vi "Z-Projection.vi"(8 "error in":errorcluster, 9 "[ROI vis]":T4 caption="[POI]" {"ROI number" min=1 format="ROI %.0f"}, 11 "Functional Imging UI Refs":T2) -> (0 "error out":errorcluster, 2 "GreenPOIMax":T1, 3 "RedPOIMax":T1)   [LabVIEW 2013]
uses:
  <vilib>/vision/Image Controls.llb/IMAQ Image.ctl
  Typedefs/ROI selector array-ROI vis.ctl
  xcontrol/Interface VIs/Interface typedefs/Interface-ROI selection cluster.ctl
  Typedefs/ROI ID Enum.ctl
  Typedefs/Functional Imging UI Refs.ctl
  xcontrol/XGrapher.xctl
  Typedefs/Groups array referecne.ctl
  Typedefs/ROI visibility mode.ctl
  Typedefs/Get-Set-Clear Control.ctl
  Typedefs/ROI parameters data type.ctl
  Global variables/gl_Functional Imaging-Global variables.vi
  <vilib>/vision/NI_Vision_Development_Module.lvlib
panel:
  out "Image 2":T1(plugin-control)
  out "Red norm max":i16
  out "Red max":i16
  out "Image":T1(plugin-control)
  out "Green norm max":i16
  in  "Normalise to approx.":i16=3000
  out "Green max":i16
  out "Multiple Z-planes added":bool
  # "[Groups] is a Typedef"
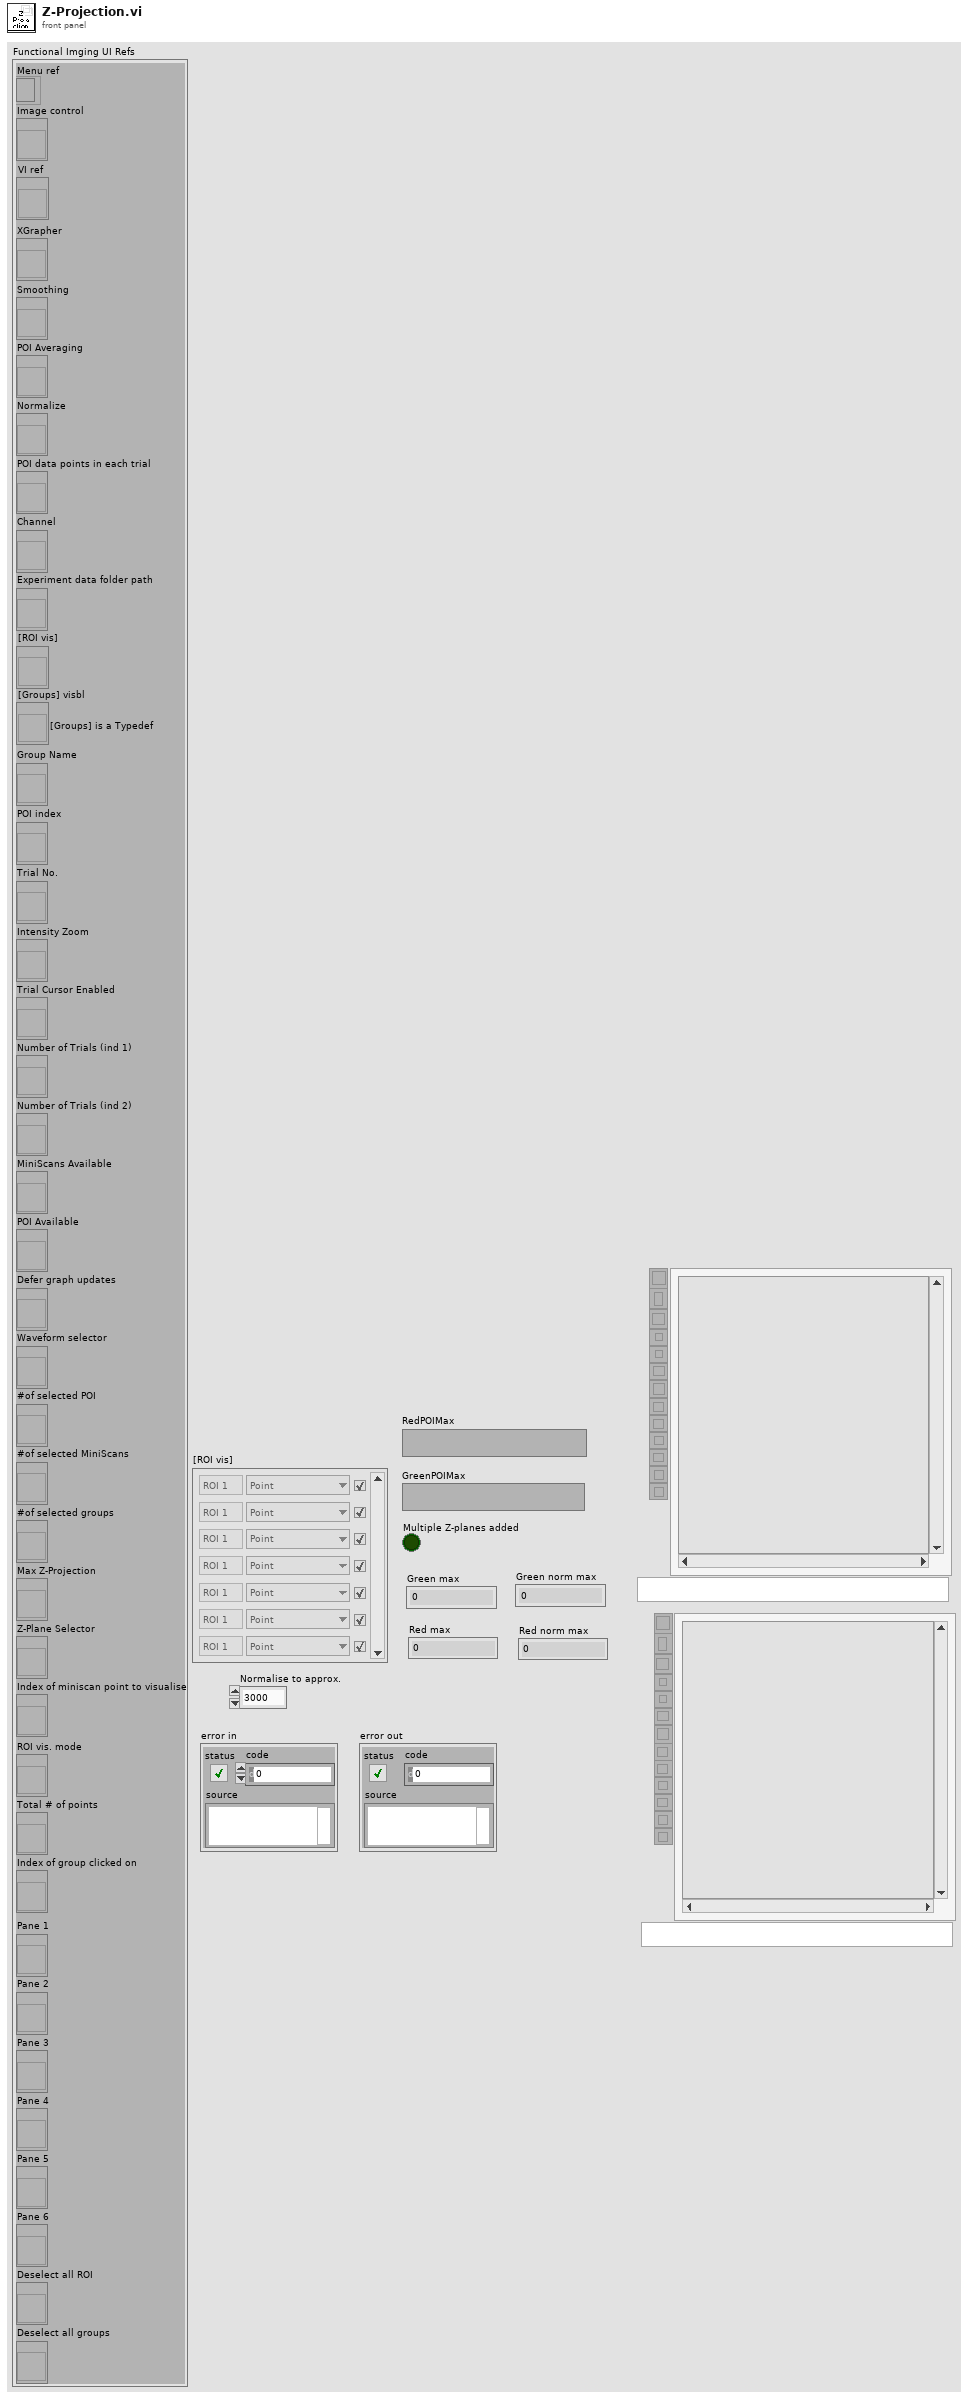
[diagram p1: front panel]
types:
  T1 = typedef "IMAQ Image.ctl" = refnum<image>
  T2 = typedef "Functional Imging UI Refs.ctl" = cluster{"Menu ref":refnum<k9>, "Image control":refnum<vi>, "VI ref":refnum<vi>, "XGrapher":refnum<vi>, "Smoothing":refnum<vi>, "POI Averaging":refnum<vi>, "Normalize":refnum<vi>, "POI data points in each trial":refnum<vi>, "Channel":refnum<vi>, "Experiment data folder path":refnum<vi>, "[ROI vis]":refnum<vi>, "[Groups] visbl":T3, "Group Name":refnum<vi>, "POI index":refnum<vi>, "Trial No.":refnum<vi>, "Intensity Zoom":refnum<vi>, "Trial Cursor Enabled":refnum<vi>, "Number of Trials (ind 1)":refnum<vi>, "Number of Trials (ind 2)":refnum<vi>, "MiniScans Available":refnum<vi>, "POI Available":refnum<vi>, "Defer graph updates":refnum<vi>, "Waveform selector":refnum<vi>, "#of selected POI":refnum<vi>, "#of selected MiniScans":refnum<vi>, "#of selected groups":refnum<vi>, "Max Z-Projection":refnum<vi>, "Z-Plane Selector":refnum<vi>, "Index of miniscan point to visualise":refnum<vi>, "ROI vis. mode":refnum<vi>, "Total # of points":refnum<vi>, "Index of group clicked on":refnum<vi>, "Pane 1":refnum<vi>, "Pane 2":refnum<vi>, "Pane 3":refnum<vi>, "Pane 4":refnum<vi>, "Pane 5":refnum<vi>, "Pane 6":refnum<vi>, "Deselect all ROI":refnum<vi>, "Deselect all groups":refnum<vi>}
  T3 = typedef "Groups array referecne.ctl" = refnum<vi>
  T4 = typedef "ROI selector array-ROI vis.ctl" = T5[]
  T5 = typedef "Interface-ROI selection cluster.ctl" = cluster{"ROI number":i32, "ROI ID":T6, "Visibility":bool}
  T6 = typedef "ROI ID Enum.ctl" = enum16{"Point", "MiniScan", "Comp. MiniScan", "Rectangle", "Comp. volume", "Arb. plane point"}
  T7 = typedef "Get-Set-Clear Control.ctl" = enum16{"Get", "Set", "Clear"}
  T8 = typedef "ROI parameters data type.ctl" = cluster{"ROI index":dbl, "ROI ID":dbl, "ROI Time (ns)":dbl, "Pixels in ROI":dbl, "X start":dbl, "Y start":dbl, "Z start":dbl, "X stop":dbl, "Y stop":dbl, "Z stop":dbl, "Angle (deg)":dbl, "Composite ID":dbl, "Number of lines":dbl, "Frame Size":dbl, "Zoom":dbl, "Laser Power (%)":dbl, "ROI group ID":dbl}
  T9 = enum32{"Average", "Min", "Max", "Clear  if < ", "Clear  if < or =", "Clear  if =", "Clear  if > or =", "Clear  if >"}
  T10 = typedef "Image Type" = u32
  T11 = typedef "Functional Parameters Cluster.ctl" = cluster{"ROI data":dbl[][], "ROI format version":i32, "Norm ROI data":dbl[][], "Norm. ROI format version":i32, "Z norm":dbl[], "Z norm format version":i32}
  T12 = typedef "Fixed strings.ctl" = cluster{"ROI file name":string, "Normalised ROI file name":string, "Zplane Pockels values file name":string, "Functional data folder name":string, "Experiment Header file name":string, "Z-stack images folder name":string, "Groups setup rel. path":string, "Groups text file rel. path":string, "TDMS files folder name (F.img)":string, "TDMS files folder name (V.acq)":string, "TDMS files folder name (Pl.acq)":string, "Cycle rel times sequence file":string, "Dynamically called VIs folder name":string, "Time Series folder base name":string}
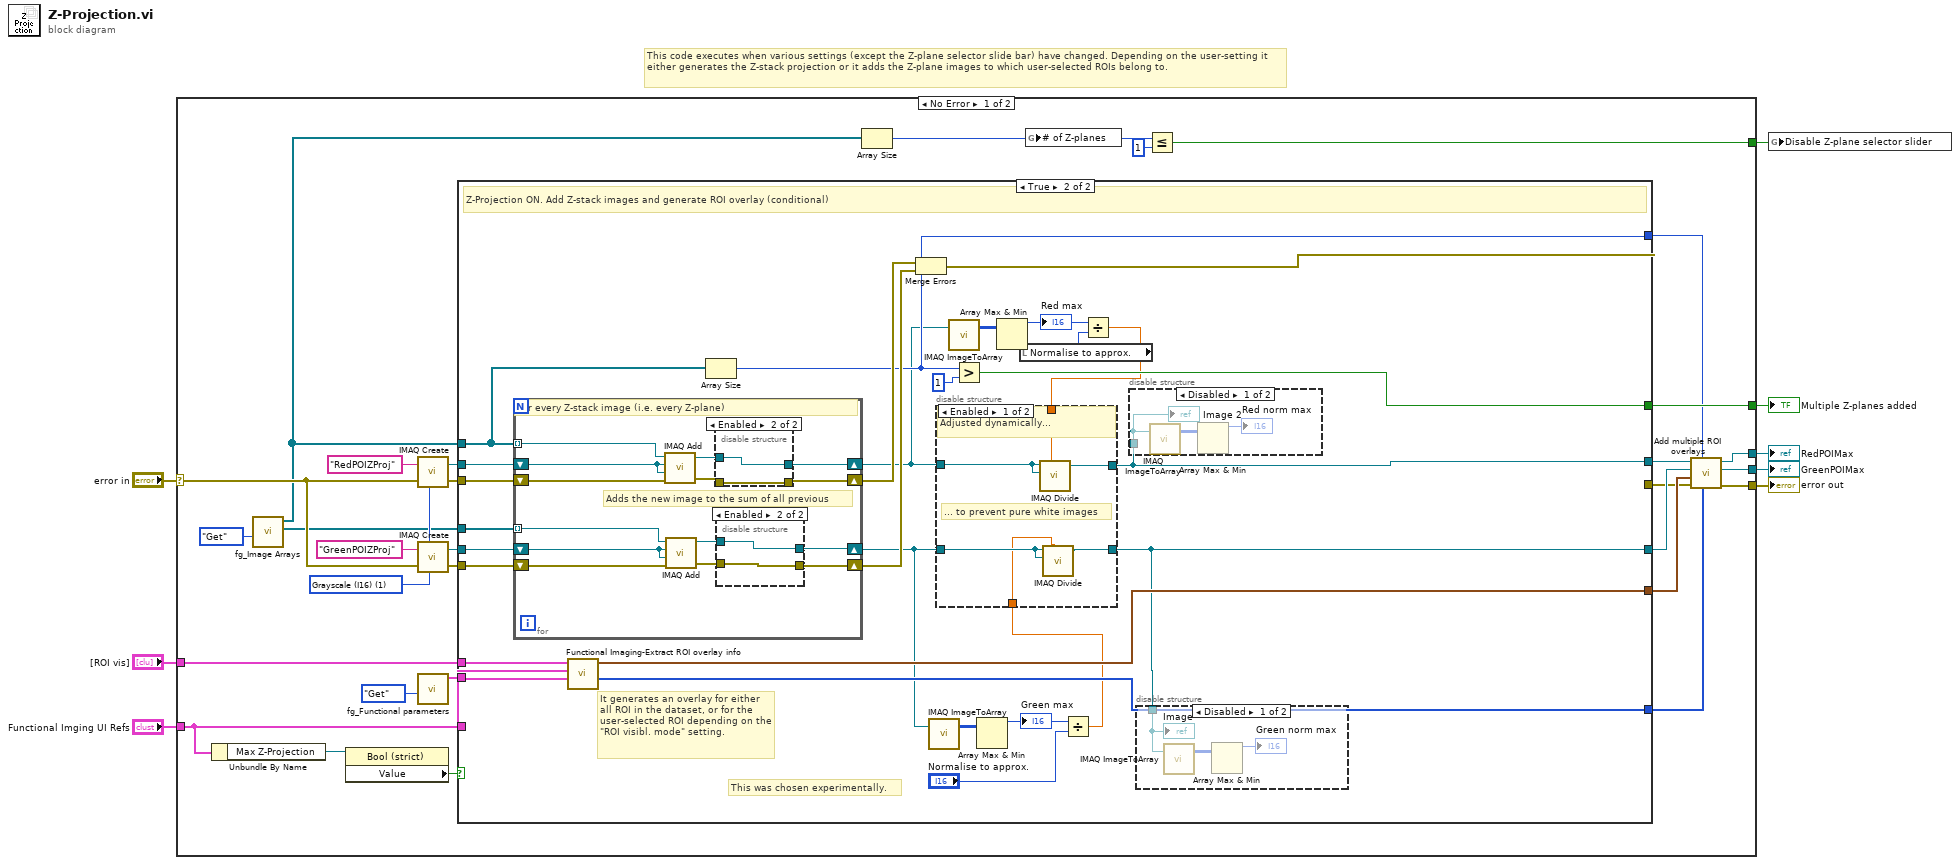
[diagram p0: block diagram]
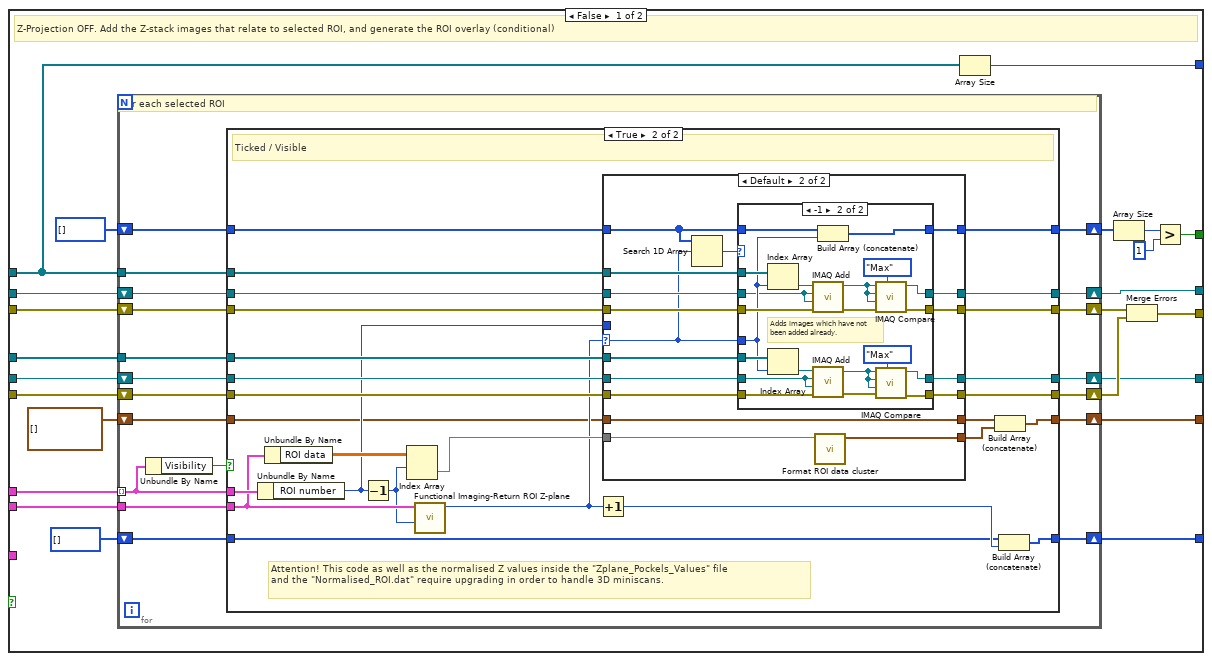
[diagram p2: hidden frame]
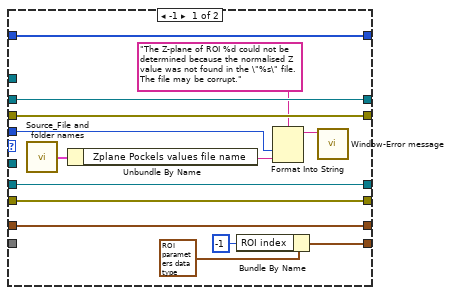
[diagram p4: hidden frame]
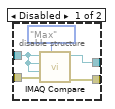
[diagram p9: hidden frame]
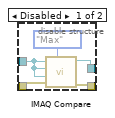
[diagram p10: hidden frame]
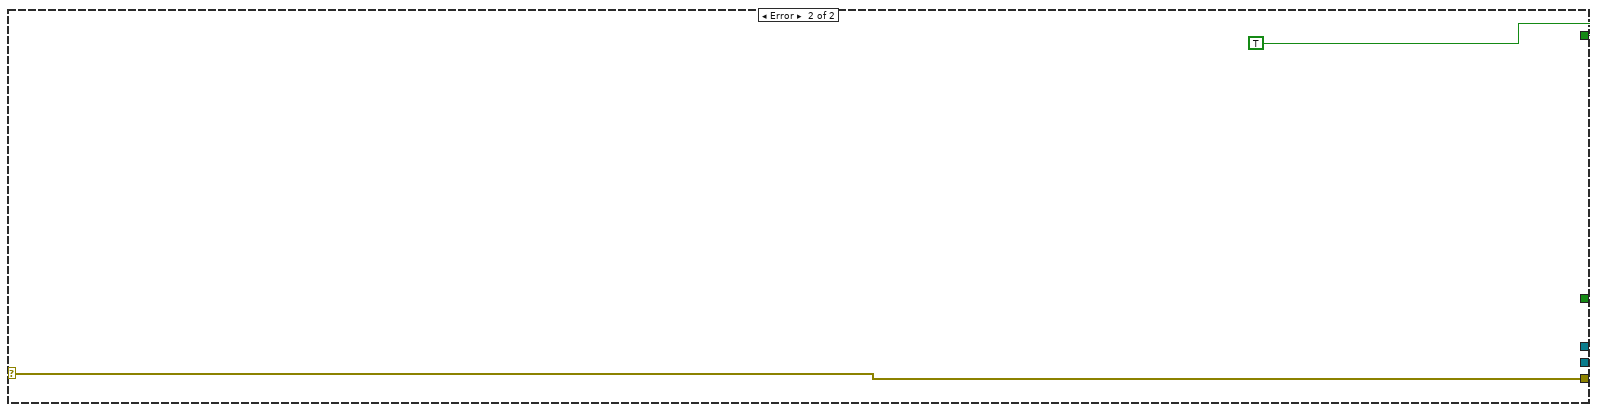
[diagram p11: hidden frame]
diagram:
  # "This code executes when various settings (except the Z-plane selector slide bar) have changed. Depending on the user-setting it either generates the Z-stack projection or it adds the Z-plane images to which user-selected ROIs belong to."
  n1 = case shown="No Error" "error in" {
    selector: "error in" -> [w31 w243]
    tunnel: "[ROI vis]" -> [w30 _]
    tunnel: [w15 _] -> w8
    tunnel: [w16 _] -> w7
    tunnel: [w11 w243] -> w6
    tunnel: [w29 _] -> w3
    tunnel: [w27 TRUE] -> w2
    tunnel: "Functional Imging UI Refs" -> [w18 _]
    frame No Error {
      w38 = T10 1 items=["Grayscale (U8)", "Grayscale (I16)", "Grayscale (SGL)", "Complex (CSG)", "RGB (U32)", "HSL (U32)", "RGB (U64)"] ("Image Type")
      n2 = Unbundle By Name(w18) -> ("Max Z-Projection"=w20:refnum<vi>)
      n3 = call "fg_Image Arrays.vi"("Function"=Get-Set-Clear_Control."Get") -> ("Green Images Array"=w21:T1[], "Red Images Array"=w22:T1[])  [unwired: 9 in]
      n4 = property on="Property Node" class="Bool (strict)"(reference=w20) -> ("Value"=w19:bool)  [unwired: 1 in, 2 out]
      n5 = call "IMAQ Create"("Image Name"="RedPOIZProj" ("string"), "Image Type"=w38, "error in (no error)"=w31) -> ("New Image"=w32:T1, "error out"=w33:errorcluster)  [unwired: 2 in]
      n6 = call "IMAQ Create"("Image Name"="GreenPOIZProj" ("string"), "Image Type"=w38, "error in (no error)"=w31) -> ("New Image"=w35:T1, "error out"=w34:errorcluster)  [unwired: 2 in]
      n7 = call "fg_Functional parameters.vi"("Function"=Get-Set-Clear_Control."Get") -> ("Functional Parameters"=w23:T11)  [unwired: 7 in, 3 out]
      n8 = case shown="True" w19 {
        tunnel: w35 -> [w61 w199]
        tunnel: w34 -> [w60 w198]
        tunnel: w33 -> [w59 w197]
        tunnel: w21 -> [w58 w196]
        tunnel: w32 -> [w57 w195]
        tunnel: [w56 w194] -> w10
        tunnel: [w39 w171] -> w17
        tunnel: [w43 w179] -> w14
        tunnel: w30 -> [w55 w186]
        tunnel: w23 -> [w52 w185]
        tunnel: w22 -> [w51 w184]
        tunnel: [w46 w190] -> w29
        tunnel: w18 -> [_ w189]
        tunnel: [w45 w183] -> w9
        tunnel: [w40 w188] -> w13
        tunnel: [w44 w187] -> w12
        frame False {
          # "Z-Projection OFF. Add the Z-stack images that relate to selected ROI, and generate the ROI overlay (conditional)"
          n9 = for {
            shift-right: [w76] -> w43
            shift-left: w61 -> [w72]
            shift-right: [w77] -> w39
            shift-left: w57 -> [w71]
            tunnel: w51 -> [w73]
            tunnel: w58 -> [w78]
            tunnel: w55 -> [w66] mode=indexing
            shift-right: [w74] -> w54
            shift-left: w59 -> [w79]
            shift-right: [w75] -> w53
            shift-left: w60 -> [w80]
            tunnel: w52 -> [w67]
            shift-right: [w69] -> w49
            shift-left: i32[] [] -> [w68]
            shift-right: [w70] -> w44
            shift-left: i32[] [] -> [w62]
            shift-right: [w63] -> w40
            shift-left: T8[] [] -> [w64]
            # "For each selected ROI"
            n10 = Unbundle By Name(w66) -> ("Visibility"=w65:bool)
            n11 = case shown="True" w65 {
              tunnel: w80 -> [w84 w113]
              tunnel: w79 -> [w83 w112]
              tunnel: w78 -> [_ w111]
              tunnel: [w82 w110] -> w77
              tunnel: [w85 w109] -> w76
              tunnel: [w84 w108] -> w75
              tunnel: [w83 w107] -> w74
              tunnel: w66 -> [_ w106]
              tunnel: w73 -> [_ w105]
              tunnel: w72 -> [w85 w103]
              tunnel: [w87 w90] -> w63
              tunnel: w71 -> [w82 w101]
              tunnel: [w86 w92] -> w70
              tunnel: [w81 w99] -> w69
              tunnel: w68 -> [w81 w98]
              tunnel: w67 -> [_ w97]
              tunnel: w64 -> [w87 w94]
              tunnel: w62 -> [w86 w91]
              frame False {
                # "Unticked / Hidden"
              }
              frame True {
                # "Attention! This code as well as the normalised Z values inside the \"Zplane_Pockels_Values\" file\nand the \"Normalised_ROI.dat\" require upgrading in order to handle 3D miniscans."
                # "Ticked / Visible"
                n12 = Unbundle By Name(w106) -> ("ROI number"=w100:i32)
                n13 = Unbundle By Name(w97) -> ("ROI data"=w102:dbl[][])
                n14 = Decrement(x=w100) -> (x-1=w96:i32)
                n15 = Index Array(array=w102, index (row)=w96) -> (element=w104:dbl[])  [unwired: 1 in]
                n16 = call "Functional Imaging-Return ROI Z-plane.vi"("ROI index (zero based)"=w96, "Functional Parameters"=w97) -> ("Zero-based index of the Z-plane the indexed ROI belongs to"=w95:i32)  [unwired: 9 in]
                n17 = Increment(x=w95) -> (x+1=w93:i32)
                n18 = case shown="Default" w95 {
                  selector: w95 -> [_ w129]
                  tunnel: w113 -> [w124 w137]
                  tunnel: w112 -> [w125 w138]
                  tunnel: w111 -> [_ w144]
                  tunnel: [w127 w143] -> w110
                  tunnel: [w126 w142] -> w109
                  tunnel: [w124 w141] -> w108
                  tunnel: [w125 w140] -> w107
                  tunnel: w105 -> [_ w139]
                  tunnel: w104 -> [_ w133]
                  tunnel: w103 -> [w126 w136]
                  tunnel: [w122 w134] -> w89
                  tunnel: w101 -> [w127 w135]
                  tunnel: w100 -> [w121 _]
                  tunnel: [w119 w132] -> w99
                  tunnel: w98 -> [w119 w131]
                  tunnel: w94 -> [w114 w128]
                  tunnel: [w114 w128] -> w88
                  frame -1 {
                    n19 = call "Source_File and folder names.vi"() -> ("Fixed strings"=w116:T12)  [unwired: 1 in]
                    n20 = Unbundle By Name(w116) -> ("Zplane Pockels values file name"=w118:string)
                    n21 = Bundle By Name(cluster=T8 {"ROI index"=0.0, "ROI ID"=0.0, "ROI Time (ns)"=0.0, "Pixels in ROI"=0.0, "X start"=0.0, "Y start"=0.0, "Z start"=0.0, "X stop"=0.0, "Y stop"=0.0, "Z stop"=0.0, "Angle (deg)"=0.0, "Composite ID"=0.0, "Number of lines"=0.0, "Frame Size"=0.0, "Zoom"=0.0, "Laser Power (%)"=0.0, "ROI group ID"=0.0} ("X-Y-Z coordinates"), "ROI index"=i64 -1) -> (w122:T8)
                    n22 = Format Into String(format string="The Z-plane of ROI %d could not be determined because the normalised Z value was not found in the \"%s\" file. The file may be corrupt." ("message"), w121, w118) -> (resulting string=w117:string)  [unwired: 2 in, 1 out]
                    n23 = call "Window-Error message.vi"("Message"=w117) -> ()  [unwired: 10 in, 1 out]
                  }
                  frame Default {
                    n24 = Search 1D Array(1D array=w131, element=w129) -> (index of element=w130:i32)  [unwired: 1 in]
                    n25 = case shown="-1" w130 {
                      tunnel: w144 -> [_ w168]
                      tunnel: [w149 w167] -> w143
                      tunnel: [w148 w166] -> w142
                      tunnel: [w146 w165] -> w141
                      tunnel: [w147 w164] -> w140
                      tunnel: w139 -> [_ w163]
                      tunnel: w129 -> [_ w152]
                      tunnel: w138 -> [w147 w162]
                      tunnel: w137 -> [w146 w161]
                      tunnel: w136 -> [w148 w159]
                      tunnel: w135 -> [w149 w150]
                      tunnel: [w145 w153] -> w132
                      tunnel: w131 -> [w145 w151]
                      frame Default {
                        # "Image already added."
                      }
                      frame -1 {
                        # "Adds images which have not\nbeen added already."
                        n26 = Index Array(array=w163, index=w152) -> (element=w155:T1)
                        n27 = Index Array(array=w168, index=w152) -> (element=w160:T1)
                        n28 = call "IMAQ Add"("Image Src A"=w155, "Image Dst"=w150, "Image Src B"=w150, "error in (no error)"=w162) -> ("Image Dst Out"=w154:T1, "error out"=w157:errorcluster)  [unwired: 3 in]
                        n29 = call "IMAQ Add"("Image Src A"=w160, "Image Dst"=w159, "Image Src B"=w159, "error in (no error)"=w161) -> ("Image Dst Out"=w158:T1, "error out"=w156:errorcluster)  [unwired: 3 in]
                        n30 = Build Array (concatenate)(w151, w152) -> (w153:i32[])
                        n31 = call "IMAQ Compare"("Operator"=T9."Max", "error in (no error)"=w157, "Image Src B"=w154, "Image Dst"=w154, "Image Src A"=w154) -> ("error out"=w164:errorcluster, "Image Dst Out"=w167:T1)  [unwired: 5 in]
                        n32 = call "IMAQ Compare"("Operator"=T9."Max", "error in (no error)"=w156, "Image Src B"=w158, "Image Dst"=w158, "Image Src A"=w158) -> ("error out"=w165:errorcluster, "Image Dst Out"=w166:T1)  [unwired: 5 in]
                      }
                    }
                    n33 = call "Format ROI data cluster.vi"("Single ROI info"=w133) -> ("X-Y-Z coordinates"=w134:T8)  [unwired: 10 in]
                  }
                }
                n34 = Build Array (concatenate)(w88, w89) -> (w90:T8[])
                n35 = Build Array (concatenate)(w91, w93) -> (w92:i32[])
              }
            }
          }
          n36 = Array Size(array=w51) -> (size(s)=w45:i32)
          n37 = Array Size(array=w49) -> (size(s)=w48:i32)
          n38 = Merge Errors(w54, w53) -> (w56:errorcluster)
          n39 = Greater?(x=w48, y=1) -> (0:w46:bool)
        }
        frame True {
          # "This was chosen experimentally."
          # "It generates an overlay for either all ROI in the dataset, or for the user-selected ROI depending on the \"ROI visibl. mode\" setting."
          # "Z-Projection ON. Add Z-stack images and generate ROI overlay (conditional)"
          n40 = for {
            shift-right: [w226] -> w178
            shift-left: w199 -> [w219]
            shift-right: [w227] -> w174
            shift-left: w195 -> [w223]
            tunnel: w184 -> [w215] mode=indexing
            tunnel: w196 -> [w214] mode=indexing
            shift-right: [w224] -> w193
            shift-left: w197 -> [w222]
            shift-right: [w225] -> w192
            shift-left: w198 -> [w218]
            # "Adds the new image to the sum of all previous"
            # "For every Z-stack image (i.e. every Z-plane)"
            n41 = call "IMAQ Add"("Image Src A"=w215, "Image Dst"=w223, "Image Src B"=w223, "error in (no error)"=w222) -> ("Image Dst Out"=w220:T1, "error out"=w221:errorcluster)  [unwired: 3 in]
            n42 = call "IMAQ Add"("Image Src A"=w214, "Image Dst"=w219, "Image Src B"=w219, "error in (no error)"=w218) -> ("Image Dst Out"=w216:T1, "error out"=w217:errorcluster)  [unwired: 3 in]
            n43 = disable-structure shown="Enabled" {
              disable-tunnel: [w239 w241] -> w227
              disable-tunnel: [w238 w240] -> w224
              disable-tunnel: w221 -> [w236 w240]
              disable-tunnel: w220 -> [w235 w241]
              frame Disabled {
                n44 = call "IMAQ Compare"("Operator"=T9."Max", "error in (no error)"=w236, "Image Src B"=w235, "Image Dst"=w235, "Image Src A"=w235) -> ("error out"=w238:errorcluster, "Image Dst Out"=w239:T1)  [unwired: 5 in]
              }
              frame Enabled {
              }
            }
            n45 = disable-structure shown="Enabled" {
              disable-tunnel: [w232 w234] -> w226
              disable-tunnel: [w231 w233] -> w225
              disable-tunnel: w217 -> [w229 w233]
              disable-tunnel: w216 -> [w228 w234]
              frame Disabled {
                n46 = call "IMAQ Compare"("Operator"=T9."Max", "error in (no error)"=w229, "Image Src B"=w228, "Image Dst"=w228, "Image Src A"=w228) -> ("error out"=w231:errorcluster, "Image Dst Out"=w232:T1)  [unwired: 5 in]
              }
              frame Enabled {
              }
            }
          }
          n47 = call "Functional Imaging-Extract ROI overlay info.vi"("Functional Imging UI Refs"=w189, "Functional Parameters"=w185, "[ROI]"=w186) -> ("[ROI index] (unity based)"=w187:i32[], "[ROI info]"=w188:T8[])  [unwired: 7 in]
          n48 = Array Size(array=w184) -> (size(s)=w183:i32)
          n49 = Merge Errors(w193, w192) -> (w194:errorcluster)
          n50 = call "IMAQ ImageToArray"("Image"=w178) -> ("Image Pixels (I16)"=w182:i16[][])  [unwired: 3 in, 4 out]
          n51 = call "IMAQ ImageToArray"("Image"=w174) -> ("Image Pixels (I16)"=w175:i16[][])  [unwired: 3 in, 4 out]
          n52 = Greater?(x=w183, y=1) -> (0:w190:bool)
          n53 = Array Max & Min(array=w182) -> (max value=w181:i16)  [unwired: 3 out]
          "Green max" <- w181
          n54 = Array Max & Min(array=w175) -> (max value=w176:i16)  [unwired: 3 out]
          "Red max" <- w176
          n55 = local read "Normalise to approx."() -> (w173:i16)
          n56 = Divide(x=w181, y="Normalise to approx.") -> (x/y=w177:dbl)
          n57 = Divide(x=w176, y=w173) -> (x/y=w172:dbl)
          n58 = disable-structure shown="Enabled" {
            disable-tunnel: [w211 w213] -> w171
            disable-tunnel: [w210 w212] -> w179
            disable-tunnel: w178 -> [w209 w212]
            disable-tunnel: w177 -> [w208 _]
            disable-tunnel: w174 -> [w207 w213]
            disable-tunnel: w172 -> [w206 _]
            frame Enabled {
              # "... to prevent pure white images"
              # "Adjusted dynamically..."
              n59 = call "IMAQ Divide"("Image Src A"=w207, "Constant"=w206, "Image Dst"=w207) -> ("Image Dst Out"=w211:T1)  [unwired: 4 in, 1 out]
              n60 = call "IMAQ Divide"("Image Src A"=w209, "Constant"=w208, "Image Dst"=w209) -> ("Image Dst Out"=w210:T1)  [unwired: 4 in, 1 out]
            }
            frame Disabled {
            }
          }
          n61 = disable-structure shown="Disabled" {
            disable-tunnel: w171 -> [w203 _]
            frame Disabled {
              n62 = call "IMAQ ImageToArray"("Image"=w203) -> ("Image Pixels (I16)"=w205:i16[][])  [unwired: 3 in, 4 out]
              n63 = Array Max & Min(array=w205) -> (max value=→"Red norm max":i16)  [unwired: 3 out]
              "Image 2" <- w203
            }
            frame Enabled {
            }
          }
          n64 = disable-structure shown="Disabled" {
            disable-tunnel: w179 -> [w200 _]
            frame Disabled {
              n65 = call "IMAQ ImageToArray"("Image"=w200) -> ("Image Pixels (I16)"=w201:i16[][])  [unwired: 3 in, 4 out]
              n66 = Array Max & Min(array=w201) -> (max value=→"Green norm max":i16)  [unwired: 3 out]
              "Image" <- w200
            }
            frame Enabled {
            }
          }
        }
      }
      n67 = Array Size(array=w22) -> (size(s)=w26:i32)
      n68 = global write "gl_Functional Imaging-Global variables.vi" "# of Z-planes"(w26) -> ()
      n69 = Less Or Equal?(x=w26, y=1) -> (x <= y?=w27:bool)
      n70 = call "Add multiple ROI overlays.vi"("[ROI index] (unity based)"=w12, "# of Z-planes"=w9, "error in"=w10, "[ROI info]"=w13, "Image 2 in"=w14, "Image 1 in"=w17) -> ("error out"=w11:errorcluster, "Image 2 out"=w15:T1, "Image 1 out"=w16:T1)  [unwired: 3 in]
    }
    frame Error {
    }
  }
  "GreenPOIMax" <- w8
  "RedPOIMax" <- w7
  "error out" <- w6
  "Multiple Z-planes added" <- w3
  n71 = global write "gl_Functional Imaging-Global variables.vi" "Disable Z-plane selector slider"(w2) -> ()
